vi "Launcher.vi"   [LabVIEW 2020]
uses:
  ErrorDaemon_class/ErrorDaemon.lvclass
  TemplateDaemon_class/TemplateDaemon.lvclass
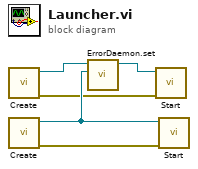
[diagram p0: block diagram]
diagram:
  n1 = call "Create.vi"() -> ("error out"=w2:errorcluster, "EventDaemon out"=w5:refnum<class "TemplateDaemon.lvclass">)  [unwired: 10 in]
  n2 = call "Create.vi"() -> ("error out"=w1:errorcluster, "EventDaemon out"=w3:refnum<class "ErrorDaemon.lvclass">)  [unwired: 10 in]
  n3 = call "ErrorDaemon.set.vi"("ErrorDaemon"=w3, "TemplateDaemon in"=w5) -> ("TemplateDaemon out"=w4:refnum<class "TemplateDaemon.lvclass">)  [unwired: 9 in]
  n4 = call-dynamic "Start.vi"("error in (no error)"=w2, "EventDaemon in"=w4) -> ()  [unwired: 8 in, 2 out]
  n5 = call-dynamic "Start.vi"("error in (no error)"=w1, "EventDaemon in"=w3) -> ()  [unwired: 8 in, 2 out]
